vi "ma_Compute Order & Cutoffs.vi"(0 "filter type":T2(ring)=enum."Bandstop", 4 "filter design":T1(ring), 5 "Gs":dbl=0.1 min=0.0 max=1.0 step=0.01 format="%0.3f", 6 "Gp":dbl=0.8 min=4.323292436654098e-306 max=2.203746971497062e-202 step=2.203746971497062e-202 format="%0.3f", 7 "fs2":dbl=0.3 step=0.1 format="%0.4f", 8 "fs1":dbl=0.2 step=0.1 format="%0.4f", 9 "fp2":dbl=0.4 step=0.1 format="%0.4f", 10 "fp1":dbl=0.1 step=0.1 format="%0.4f") -> (1 "N":i32=5, 2 "fh":dbl=0.3866728697205381 format="%0.4f", 3 "fl":dbl=0.10344661633206745 format="%0.4f")   [LabVIEW 2020, in "NI_MAPro.lvlib"]
uses:
  NI_MAPro.lvlib
panel:
  out "?":cluster{cluster{dbl, dbl}[]}[](graph)=[{[{0.0, 0.8}, {0.1, 0.8}]}, {[{0.2, 0.1}, {0.3, 0.1}]}, {[{0.4, 0.8}, {0.5, 0.8}]}, {[]}, {[{0.10344661633206745, -inf}, {0.10344661633206745, inf}, {0.3866728697205381, inf}, {0.3866728697205381, -inf}]}]
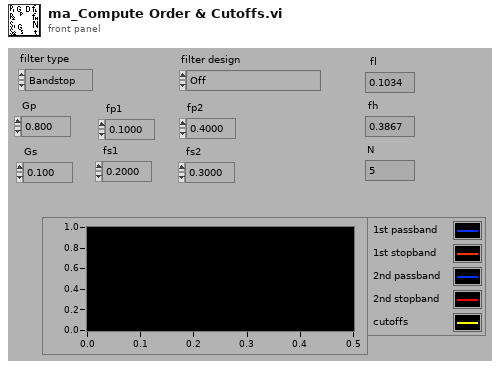
[diagram p1: front panel]
types:
  T1 = enum32{"Off", "Butterworth", "Chebyshev", "Inverse Chebyshev", "Elliptic", "Bessel"}
  T2 = enum32{"Lowpass", "Highpass", "Bandpass", "Bandstop"}
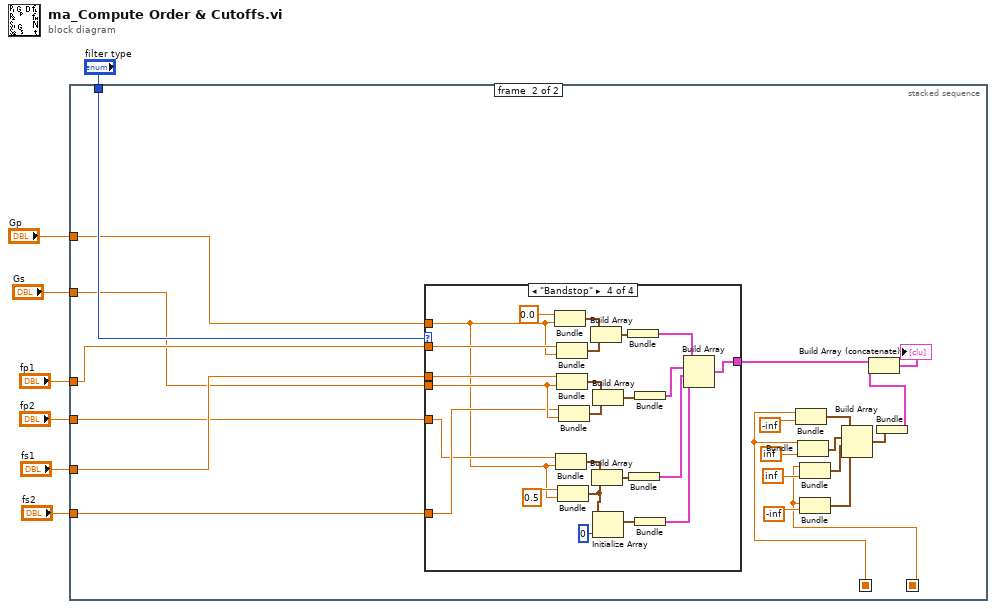
[diagram p0: block diagram]
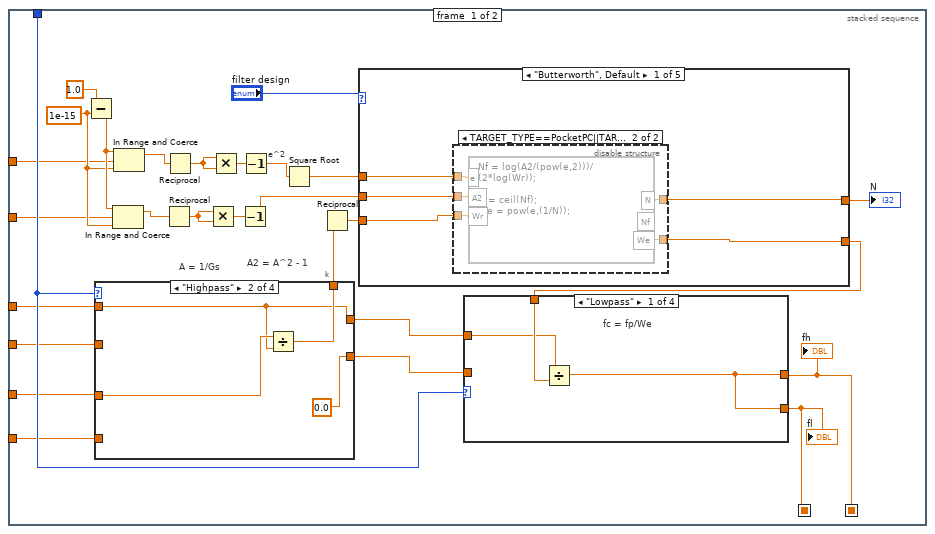
[diagram p2: hidden frame]
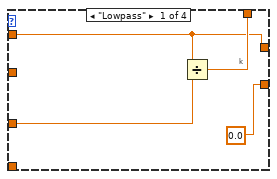
[diagram p3: hidden frame]
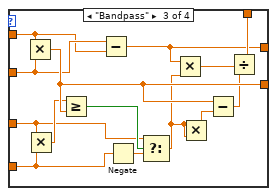
[diagram p4: hidden frame]
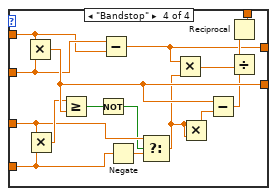
[diagram p5: hidden frame]
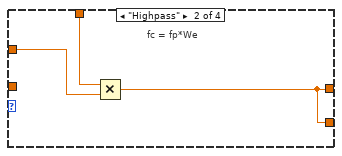
[diagram p6: hidden frame]
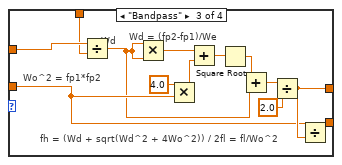
[diagram p7: hidden frame]
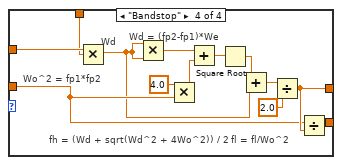
[diagram p8: hidden frame]
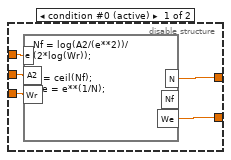
[diagram p9: hidden frame]
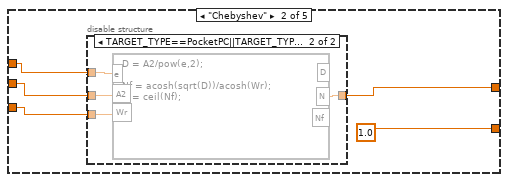
[diagram p10: hidden frame]
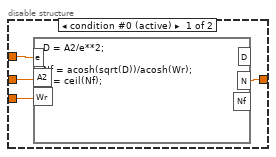
[diagram p11: hidden frame]
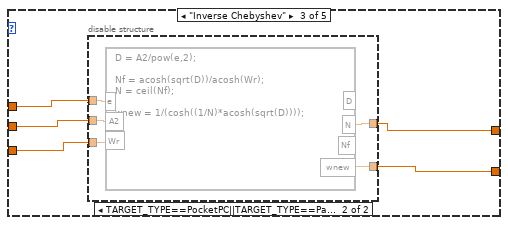
[diagram p12: hidden frame]
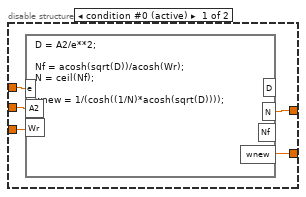
[diagram p13: hidden frame]
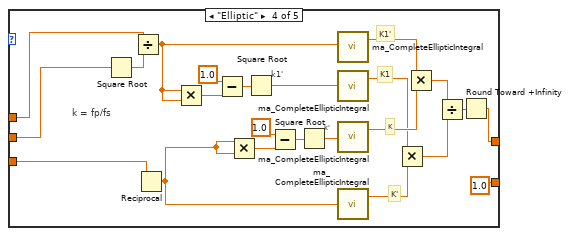
[diagram p14: hidden frame]
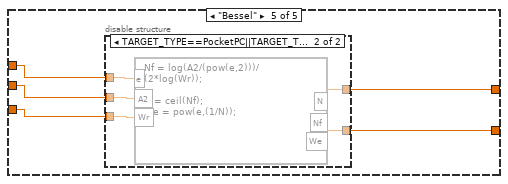
[diagram p15: hidden frame]
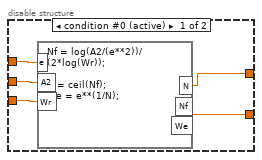
[diagram p16: hidden frame]
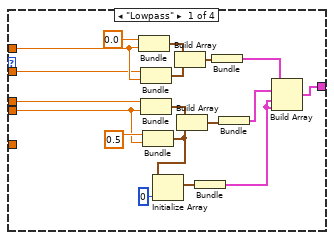
[diagram p17: hidden frame]
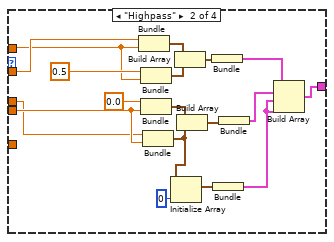
[diagram p18: hidden frame]
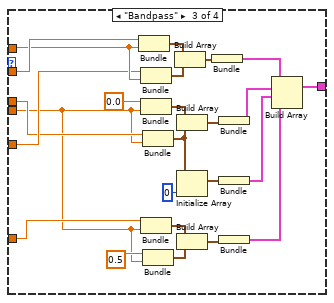
[diagram p19: hidden frame]
diagram:
  n1 = stacked-sequence {
    seq-local: [w22 _] -> [_ w194]
    seq-local: [w23 _] -> [_ w195]
    tunnel: "filter type" -> [w14 w193]
    tunnel: "Gp" -> [w13 w192]
    tunnel: "Gs" -> [w12 w189]
    tunnel: "fp1" -> [w11 w191]
    tunnel: "fp2" -> [w10 w188]
    tunnel: "fs1" -> [w9 w190]
    tunnel: "fs2" -> [w8 w187]
    frame #0 {
      w18 = 1e-15
      # "e^2"
      # "A = 1/Gs"
      # "A2 = A^2 - 1"
      # "k"
      n2 = Subtract(x=1.0, y=w18) -> (x-y=w19:dbl)
      n3 = case shown="\"Highpass\"" w14 {
        tunnel: [w39 w43 w56 w58] -> w31
        tunnel: [w36 w40 w55 w71] -> w30
        tunnel: [0.0 0.0 w54 w70] -> w29
        tunnel: w10 -> [_ _ w53 w69]
        tunnel: w11 -> [w36 w40 w52 w68]
        tunnel: w9 -> [w38 w41 w50 w66]
        tunnel: w8 -> [_ _ w44 w60]
        frame "Lowpass" {
          # "k"
          n4 = Divide(x=w36, y=w38) -> (x/y=w39:dbl)
        }
        frame "Highpass" {
          n5 = Divide(x=w41, y=w40) -> (x/y=w43:dbl)
        }
        frame "Bandpass" {
          n6 = Multiply(x=w52, y=w53) -> (x*y=w54:dbl)
          n7 = Multiply(x=w50, y=w44) -> (x*y=w51:dbl)
          n8 = Greater Or Equal?(x=w51, y=w54) -> (x >= y?=w57:bool)
          n9 = Subtract(x=w53, y=w52) -> (x-y=w55:dbl)
          n10 = Negate(x=w44) -> (-x=w49:dbl)
          n11 = Select(t=w50, s=w57, f=w49) -> (s? t:f=w48:dbl)
          n12 = Multiply(x=w55, y=w48) -> (x*y=w45:dbl)
          n13 = Multiply(x=w48, y=w48) -> (x*y=w47:dbl)
          n14 = Subtract(x=w54, y=w47) -> (x-y=w46:dbl)
          n15 = Divide(x=w45, y=w46) -> (x/y=w56:dbl)
        }
        frame "Bandstop" {
          n16 = Multiply(x=w68, y=w69) -> (x*y=w70:dbl)
          n17 = Multiply(x=w66, y=w60) -> (x*y=w67:dbl)
          n18 = Greater Or Equal?(x=w67, y=w70) -> (x >= y?=w73:bool)
          n19 = Not(x=w73) -> (.not. x?=w59:bool)
          n20 = Subtract(x=w69, y=w68) -> (x-y=w71:dbl)
          n21 = Negate(x=w60) -> (-x=w65:dbl)
          n22 = Select(t=w66, s=w59, f=w65) -> (s? t:f=w64:dbl)
          n23 = Multiply(x=w71, y=w64) -> (x*y=w61:dbl)
          n24 = Multiply(x=w64, y=w64) -> (x*y=w63:dbl)
          n25 = Subtract(x=w70, y=w63) -> (x-y=w62:dbl)
          n26 = Divide(x=w61, y=w62) -> (x/y=w72:dbl)
          n27 = Reciprocal(x=w72) -> (1/x=w58:dbl)
        }
      }
      n28 = In Range and Coerce(upper limit=w19, x=w12, lower limit=w18) -> (coerced(x)=w17:dbl)  [unwired: 1 out]
      n29 = In Range and Coerce(upper limit=w19, x=w13, lower limit=w18) -> (coerced(x)=w16:dbl)  [unwired: 1 out]
      n30 = Reciprocal(x=w17) -> (1/x=w34:dbl)
      n31 = Reciprocal(x=w16) -> (1/x=w24:dbl)
      n32 = Multiply(x=w34, y=w34) -> (x*y=w33:dbl)
      n33 = Multiply(x=w24, y=w24) -> (x*y=w25:dbl)
      n34 = Decrement(x=w33) -> (x-1=w35:dbl)
      n35 = Decrement(x=w25) -> (x-1=w26:dbl)
      n36 = Square Root(x=w26) -> (sqrt(x)=w27:dbl)
      n37 = Reciprocal(x=w31) -> (1/x=w32:dbl)
      n38 = case shown="\"Butterworth\", Default" "filter design" {
        tunnel: w32 -> [w110 w124 w137 w150 w176]
        tunnel: [w109 1.0 w134 1.0 w175] -> w28
        tunnel: w27 -> [w108 w123 w136 w153 w174]
        tunnel: [w106 w122 w135 w152 w173] -> w15
        tunnel: w35 -> [w107 w125 w138 w149 w172]
        frame "Butterworth", Default {
          n39 = disable-structure shown="TARGET_TYPE==PocketPC||TARGET_TYPE==PalmOS||TARGET_TYPE==Embedded" {
            disable-tunnel: w110 -> [w115 w120]
            disable-tunnel: [w114 w119] -> w109
            disable-tunnel: w108 -> [w113 w118]
            disable-tunnel: w107 -> [w112 w117]
            disable-tunnel: [w111 w116] -> w106
            frame condition #0 (active) {
              n40 = formula code="Nf = log(A2/(e**2))/\n(2*log(Wr));\n\nN = ceil(Nf);\nWe = e**(1/N);"("e"=w113, "A2"=w112, "Wr"=w115) -> ("N"=w111:dbl, "We"=w114:dbl)  [unwired: 1 out]
            }
            frame condition #1 {
              n41 = formula code="Nf = log(A2/(pow(e,2)))/\n(2*log(Wr));\n\nN = ceil(Nf);\nWe = pow(e,(1/N));"("e"=w118, "A2"=w117, "Wr"=w120) -> ("N"=w116:dbl, "We"=w119:dbl)  [unwired: 1 out]
            }
          }
        }
        frame "Chebyshev" {
          n42 = disable-structure shown="TARGET_TYPE==PocketPC||TARGET_TYPE==PalmOS||TARGET_TYPE==Embedded" {
            disable-tunnel: w125 -> [w129 w133]
            disable-tunnel: w124 -> [w128 w132]
            disable-tunnel: w123 -> [w127 w131]
            disable-tunnel: [w126 w130] -> w122
            frame condition #0 (active) {
              n43 = formula code="D = A2/e**2;\n\nNf = acosh(sqrt(D))/acosh(Wr);\nN = ceil(Nf);"("e"=w127, "A2"=w129, "Wr"=w128) -> ("N"=w126:dbl)  [unwired: 2 out]
            }
            frame condition #1 {
              n44 = formula code="D = A2/pow(e,2);\n\nNf = acosh(sqrt(D))/acosh(Wr);\nN = ceil(Nf);"("e"=w131, "A2"=w133, "Wr"=w132) -> ("N"=w130:dbl)  [unwired: 2 out]
            }
          }
        }
        frame "Inverse Chebyshev" {
          n45 = disable-structure shown="TARGET_TYPE==PocketPC||TARGET_TYPE==PalmOS||TARGET_TYPE==Embedded" {
            disable-tunnel: w138 -> [w143 w148]
            disable-tunnel: w137 -> [w142 w147]
            disable-tunnel: w136 -> [w141 w146]
            disable-tunnel: [w140 w145] -> w135
            disable-tunnel: [w139 w144] -> w134
            frame condition #0 (active) {
              n46 = formula code="D = A2/e**2;\n\nNf = acosh(sqrt(D))/acosh(Wr);\nN = ceil(Nf);\n\nwnew = 1/(cosh((1/N)*acosh(sqrt(D))));"("e"=w141, "A2"=w143, "Wr"=w142) -> ("N"=w140:dbl, "wnew"=w139:dbl)  [unwired: 2 out]
            }
            frame condition #1 {
              n47 = formula code="D = A2/pow(e,2);\n\nNf = acosh(sqrt(D))/acosh(Wr);\nN = ceil(Nf);\n\nwnew = 1/(cosh((1/N)*acosh(sqrt(D))));"("e"=w146, "A2"=w148, "Wr"=w147) -> ("N"=w145:dbl, "wnew"=w144:dbl)  [unwired: 2 out]
            }
          }
        }
        frame "Elliptic" {
          # "K1"
          # "k1'"
          # "K'"
          # "K1'"
          # "K"
          # "k'"
          # "k = fp/fs"
          n48 = Square Root(x=w149) -> (sqrt(x)=w171:dbl)
          n49 = Divide(x=w153, y=w171) -> (x/y=w163:dbl)
          n50 = Reciprocal(x=w150) -> (1/x=w154:dbl)
          n51 = Multiply(x=w163, y=w163) -> (x*y=w165:dbl)
          n52 = Subtract(x=1.0, y=w165) -> (x-y=w166:dbl)
          n53 = Multiply(x=w154, y=w154) -> (x*y=w169:dbl)
          n54 = Square Root(x=w166) -> (sqrt(x)=w162:dbl)
          n55 = Subtract(x=1.0, y=w169) -> (x-y=w168:dbl)
          n56 = Square Root(x=w168) -> (sqrt(x)=w167:dbl)
          n57 = call "ma_CompleteEllipticIntegral.vi"("k'"=w163) -> ("cei(k)"=w161:dbl)  [unwired: 1 out]
          n58 = call "ma_CompleteEllipticIntegral.vi"("k'"=w162) -> ("cei(k)"=w155:dbl)  [unwired: 1 out]
          n59 = call "ma_CompleteEllipticIntegral.vi"("k'"=w167) -> ("cei(k)"=w160:dbl)  [unwired: 1 out]
          n60 = call "ma_CompleteEllipticIntegral.vi"("k'"=w154) -> ("cei(k)"=w159:dbl)  [unwired: 1 out]
          n61 = Multiply(x=w155, y=w159) -> (x*y=w158:dbl)
          n62 = Multiply(x=w161, y=w160) -> (x*y=w157:dbl)
          n63 = Divide(x=w157, y=w158) -> (x/y=w156:dbl)
          n64 = Round Toward +Infinity(x=w156) -> (ceil(x): smallest int >= x=w152:dbl)
        }
        frame "Bessel" {
          n65 = disable-structure shown="TARGET_TYPE==PocketPC||TARGET_TYPE==PalmOS||TARGET_TYPE==Embedded" {
            disable-tunnel: w176 -> [w181 w186]
            disable-tunnel: [w180 w185] -> w175
            disable-tunnel: w174 -> [w179 w184]
            disable-tunnel: [w178 w183] -> w173
            disable-tunnel: w172 -> [w177 w182]
            frame condition #0 (active) {
              n66 = formula code="Nf = log(A2/(e**2))/\n(2*log(Wr));\n\nN = ceil(Nf);\nWe = e**(1/N);"("e"=w179, "A2"=w177, "Wr"=w181) -> ("N"=w178:dbl, "We"=w180:dbl)  [unwired: 1 out]
            }
            frame condition #1 {
              n67 = formula code="Nf = log(A2/(pow(e,2)))/\n(2*log(Wr));\n\nN = ceil(Nf);\nWe = pow(e,(1/N));"("e"=w184, "A2"=w182, "Wr"=w186) -> ("N"=w183:dbl, "We"=w185:dbl)  [unwired: 1 out]
            }
          }
        }
      }
      "N" <- w15
      n68 = case shown="\"Lowpass\"" w14 {
        tunnel: [w74 w77 w92 w105] -> w23
        tunnel: [w74 w77 w91 w104] -> w22
        tunnel: w30 -> [w75 w78 w90 w103]
        tunnel: w29 -> [_ _ w89 w102]
        tunnel: w28 -> [w76 w79 w82 w95]
        frame "Lowpass" {
          # "fc = fp/We"
          n69 = Divide(x=w75, y=w76) -> (x/y=w74:dbl)
        }
        frame "Highpass" {
          # "fc = fp*We"
          n70 = Multiply(x=w79, y=w78) -> (x*y=w77:dbl)
        }
        frame "Bandpass" {
          # "fh = (Wd + sqrt(Wd^2 + 4Wo^2)) / 2"
          # "Wd = (fp2-fp1)/We"
          # "Wo^2 = fp1*fp2"
          # "Wd"
          # "fl = fl/Wo^2"
          n71 = Divide(x=w90, y=w82) -> (x/y=w80:dbl)
          n72 = Multiply(x=w80, y=w80) -> (x*y=w81:dbl)
          n73 = Multiply(x=4.0, y=w89) -> (x*y=w84:dbl)
          n74 = Add(x=w81, y=w84) -> (x+y=w85:dbl)
          n75 = Square Root(x=w85) -> (sqrt(x)=w86:dbl)
          n76 = Add(x=w86, y=w80) -> (x+y=w87:dbl)
          n77 = Divide(x=w87, y=2.0) -> (x/y=w91:dbl)
          n78 = Divide(x=w89, y=w91) -> (x/y=w92:dbl)
        }
        frame "Bandstop" {
          # "fh = (Wd + sqrt(Wd^2 + 4Wo^2)) / 2"
          # "Wd = (fp2-fp1)*We"
          # "Wo^2 = fp1*fp2"
          # "Wd"
          # "fl = fl/Wo^2"
          n79 = Multiply(x=w103, y=w95) -> (x*y=w93:dbl)
          n80 = Multiply(x=w93, y=w93) -> (x*y=w94:dbl)
          n81 = Multiply(x=4.0, y=w102) -> (x*y=w97:dbl)
          n82 = Add(x=w94, y=w97) -> (x+y=w98:dbl)
          n83 = Square Root(x=w98) -> (sqrt(x)=w99:dbl)
          n84 = Add(x=w99, y=w93) -> (x+y=w100:dbl)
          n85 = Divide(x=w100, y=2.0) -> (x/y=w104:dbl)
          n86 = Divide(x=w102, y=w104) -> (x/y=w105:dbl)
        }
      }
      "fh" <- w22
      "fl" <- w23
    }
    frame #1 {
      n87 = case shown="\"Bandstop\"" w193 {
        tunnel: [w216 w234 w259 w282] -> w196
        tunnel: w192 -> [w211 w228 w248 w268]
        tunnel: w191 -> [w210 w229 w249 w273]
        tunnel: w190 -> [w209 w226 w246 w272]
        tunnel: w189 -> [w208 w227 w244 w271]
        tunnel: w188 -> [_ _ w247 w269]
        tunnel: w187 -> [_ _ w245 w270]
        frame "Lowpass" {
          n88 = Bundle(0.0, "Gp"=w211) -> (w224:cluster{dbl, "Gp":dbl})  [unwired: 1 in]
          n89 = Bundle("fp1"=w210, "Gp"=w211) -> (w223:cluster{"fp1":dbl, "Gp":dbl})  [unwired: 1 in]
          n90 = Bundle("fs1"=w209, "Gs"=w208) -> (w222:cluster{"fs1":dbl, "Gs":dbl})  [unwired: 1 in]
          n91 = Bundle(0.5, "Gs"=w208) -> (w213:cluster{dbl, "Gs":dbl})  [unwired: 1 in]
          n92 = Initialize Array(w213, 0) -> (w215:cluster{dbl, "Gs":dbl}[])
          n93 = Build Array(w224, w223) -> (w220:cluster{"fp1":dbl, "Gp":dbl}[])
          n94 = Build Array(w222, w213) -> (w218:cluster{"fs1":dbl, "Gs":dbl}[])
          n95 = Bundle(w215) -> (w212:cluster{cluster{dbl, "Gs":dbl}[]})  [unwired: 1 in]
          n96 = Bundle(w220) -> (w219:cluster{cluster{"fp1":dbl, "Gp":dbl}[]})  [unwired: 1 in]
          n97 = Bundle(w218) -> (w217:cluster{cluster{"fs1":dbl, "Gs":dbl}[]})  [unwired: 1 in]
          n98 = Build Array(w219, w217, w212, w212) -> (w216:cluster{cluster{"fs1":dbl, "Gs":dbl}[]}[])
        }
        frame "Highpass" {
          n99 = Bundle("fp1"=w229, "Gp"=w228) -> (w243:cluster{"fp1":dbl, "Gp":dbl})  [unwired: 1 in]
          n100 = Bundle(0.5, "Gp"=w228) -> (w242:cluster{dbl, "Gp":dbl})  [unwired: 1 in]
          n101 = Bundle(0.0, "Gs"=w227) -> (w241:cluster{dbl, "Gs":dbl})  [unwired: 1 in]
          n102 = Bundle("fs1"=w226, "Gs"=w227) -> (w231:cluster{"fs1":dbl, "Gs":dbl})  [unwired: 1 in]
          n103 = Initialize Array(w231, 0) -> (w233:cluster{"fs1":dbl, "Gs":dbl}[])
          n104 = Build Array(w243, w242) -> (w240:cluster{"fp1":dbl, "Gp":dbl}[])
          n105 = Build Array(w241, w231) -> (w238:cluster{"fs1":dbl, "Gs":dbl}[])
          n106 = Bundle(w240) -> (w239:cluster{cluster{"fp1":dbl, "Gp":dbl}[]})  [unwired: 1 in]
          n107 = Bundle(w233) -> (w230:cluster{cluster{"fs1":dbl, "Gs":dbl}[]})  [unwired: 1 in]
          n108 = Bundle(w238) -> (w237:cluster{cluster{"fs1":dbl, "Gs":dbl}[]})  [unwired: 1 in]
          n109 = Build Array(w239, w237, w230, w230) -> (w234:cluster{cluster{"fs1":dbl, "Gs":dbl}[]}[])
        }
        frame "Bandpass" {
          n110 = Bundle("fp1"=w249, "Gp"=w248) -> (w267:cluster{"fp1":dbl, "Gp":dbl})  [unwired: 1 in]
          n111 = Bundle("fp2"=w247, "Gp"=w248) -> (w266:cluster{"fp2":dbl, "Gp":dbl})  [unwired: 1 in]
          n112 = Bundle(0.0, "Gs"=w244) -> (w265:cluster{dbl, "Gs":dbl})  [unwired: 1 in]
          n113 = Bundle("fs2"=w245, "Gs"=w244) -> (w250:cluster{"fs2":dbl, "Gs":dbl})  [unwired: 1 in]
          n114 = Bundle("fs1"=w246, "Gs"=w244) -> (w252:cluster{"fs1":dbl, "Gs":dbl})  [unwired: 1 in]
          n115 = Bundle(0.5, "Gs"=w244) -> (w254:cluster{dbl, "Gs":dbl})  [unwired: 1 in]
          n116 = Build Array(w267, w266) -> (w264:cluster{"fp2":dbl, "Gp":dbl}[])
          n117 = Build Array(w265, w252) -> (w262:cluster{"fs1":dbl, "Gs":dbl}[])
          n118 = Initialize Array(w252, 0) -> (w258:cluster{"fs1":dbl, "Gs":dbl}[])
          n119 = Build Array(w250, w254) -> (w256:cluster{"fs2":dbl, "Gs":dbl}[])
          n120 = Bundle(w264) -> (w263:cluster{cluster{"fp2":dbl, "Gp":dbl}[]})  [unwired: 1 in]
          n121 = Bundle(w262) -> (w261:cluster{cluster{"fs1":dbl, "Gs":dbl}[]})  [unwired: 1 in]
          n122 = Bundle(w258) -> (w257:cluster{cluster{"fs1":dbl, "Gs":dbl}[]})  [unwired: 1 in]
          n123 = Bundle(w256) -> (w253:cluster{cluster{"fs2":dbl, "Gs":dbl}[]})  [unwired: 1 in]
          n124 = Build Array(w263, w261, w257, w253) -> (w259:cluster{cluster{"fs2":dbl, "Gs":dbl}[]}[])
        }
        frame "Bandstop" {
          n125 = Bundle(0.0, "Gp"=w268) -> (w290:cluster{dbl, "Gp":dbl})  [unwired: 1 in]
          n126 = Bundle("fp2"=w269, "Gp"=w268) -> (w280:cluster{"fp2":dbl, "Gp":dbl})  [unwired: 1 in]
          n127 = Bundle("fp1"=w273, "Gp"=w268) -> (w289:cluster{"fp1":dbl, "Gp":dbl})  [unwired: 1 in]
          n128 = Bundle("fs1"=w272, "Gs"=w271) -> (w287:cluster{"fs1":dbl, "Gs":dbl})  [unwired: 1 in]
          n129 = Bundle(0.5, "Gp"=w268) -> (w275:cluster{dbl, "Gp":dbl})  [unwired: 1 in]
          n130 = Bundle("fs2"=w270, "Gs"=w271) -> (w288:cluster{"fs2":dbl, "Gs":dbl})  [unwired: 1 in]
          n131 = Build Array(w290, w289) -> (w286:cluster{"fp1":dbl, "Gp":dbl}[])
          n132 = Build Array(w280, w275) -> (w281:cluster{"fp2":dbl, "Gp":dbl}[])
          n133 = Build Array(w287, w288) -> (w284:cluster{"fs2":dbl, "Gs":dbl}[])
          n134 = Initialize Array(w275, 0) -> (w277:cluster{dbl, "Gp":dbl}[])
          n135 = Bundle(w286) -> (w285:cluster{cluster{"fp1":dbl, "Gp":dbl}[]})  [unwired: 1 in]
          n136 = Bundle(w281) -> (w278:cluster{cluster{"fp2":dbl, "Gp":dbl}[]})  [unwired: 1 in]
          n137 = Bundle(w284) -> (w283:cluster{cluster{"fs2":dbl, "Gs":dbl}[]})  [unwired: 1 in]
          n138 = Bundle(w277) -> (w274:cluster{cluster{dbl, "Gp":dbl}[]})  [unwired: 1 in]
          n139 = Build Array(w285, w283, w278, w274) -> (w282:cluster{cluster{"fp2":dbl, "Gp":dbl}[]}[])
        }
      }
      n140 = Bundle(w195, -inf) -> (w199:cluster{dbl, dbl})  [unwired: 1 in]
      n141 = Bundle(w195, inf) -> (w205:cluster{dbl, dbl})  [unwired: 1 in]
      n142 = Bundle(w194, inf) -> (w206:cluster{dbl, dbl})  [unwired: 1 in]
      n143 = Bundle(w194, -inf) -> (w207:cluster{dbl, dbl})  [unwired: 1 in]
      n144 = Build Array(w199, w205, w206, w207) -> (w198:cluster{dbl, dbl}[])
      n145 = Bundle(w198) -> (w200:cluster{cluster{dbl, dbl}[]})  [unwired: 1 in]
      n146 = Build Array (concatenate)(w196, w200) -> (→"?":cluster{cluster{"fp2":dbl, "Gp":dbl}[]}[])
    }
  }
